vi "Query Temperature.vi"(8 "error in (no error)":errorcluster, 11 "VISA resource name":refnum<visa-resource-name>) -> (0 "error out":errorcluster, 1 "Ch2 Temp (C)":i32(slide) scale=0.0..150.0, 2 "Ch1 Temp (C)":i32(slide) scale=0.0..150.0, 3 "VISA resource name out":refnum<visa-resource-name>, 4 "IC Temp (C)":i32(slide) scale=0.0..150.0, 5 "Temps":T1 {"IC Temp (C)" scale=0.0..150.0; "Ch2 Temp (C)" scale=0.0..150.0; "Ch1 Temp (C)" scale=0.0..150.0})   [LabVIEW 2012, in "Roboteq.lvlib"]
uses:
  Roboteq.lvlib
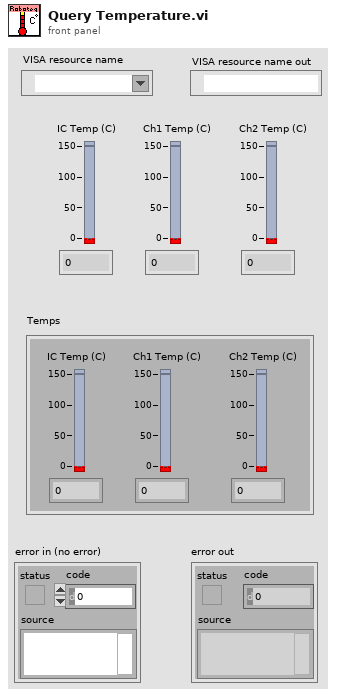
[diagram p1: front panel]
types:
  T1 = cluster{"Ch1 Temp (C)":i32, "Ch2 Temp (C)":i32, "IC Temp (C)":i32}
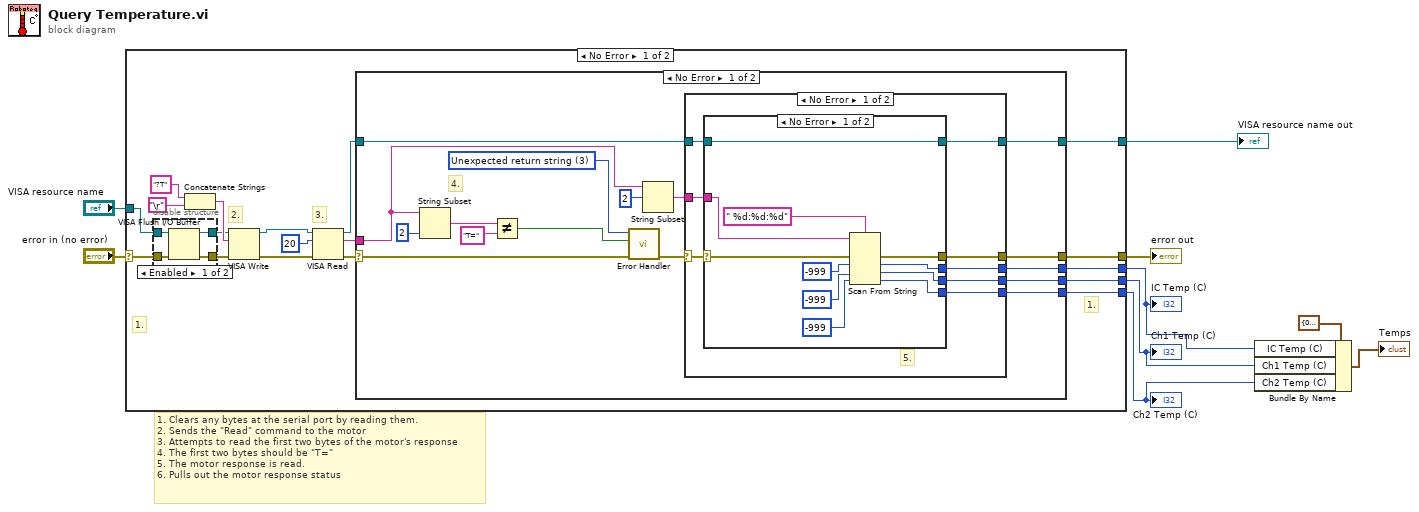
[diagram p0: block diagram]
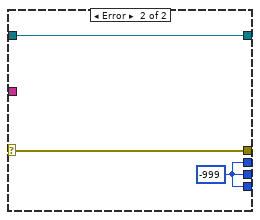
[diagram p3: hidden frame]
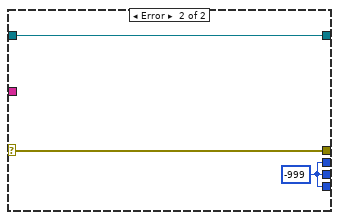
[diagram p4: hidden frame]
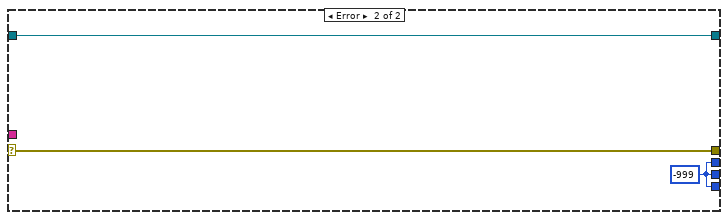
[diagram p5: hidden frame]
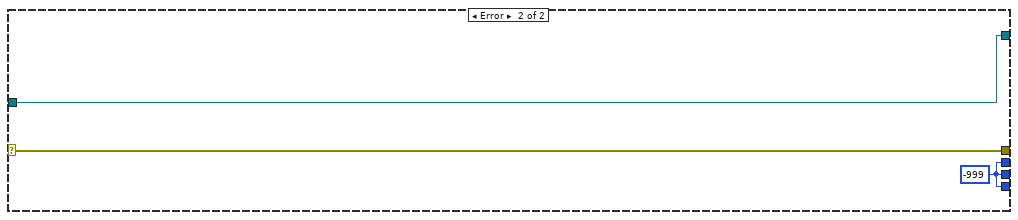
[diagram p6: hidden frame]
diagram:
  # "1. Clears any bytes at the serial port by reading them.\n2. Sends the \"Read\" command to the motor\n3. Attempts to read the first two bytes of the motor's response\n4. The first two bytes should be \"T=\"\n5. The motor response is read.\n6. Pulls out the motor response status"
  n1 = case shown="No Error" "error in (no error)" {
    selector: "error in (no error)" -> [w12 w80]
    tunnel: [w15 w80] -> w8
    tunnel: [w17 w79] -> w2
    tunnel: [w16 w79] -> w1
    tunnel: [w18 w79] -> w3
    tunnel: "VISA resource name" -> [w13 w78]
    tunnel: [w14 w78] -> w6
    frame No Error {
      # "1."
      # "3."
      # "2."
      # "1."
      n2 = disable-structure shown="Enabled" {
        disable-tunnel: w13 -> [w31 w33]
        disable-tunnel: w12 -> [w30 w32]
        disable-tunnel: [w29 w32] -> w11
        disable-tunnel: [w28 w33] -> w10
        frame Enabled {
          n3 = VISA Flush I/O Buffer(VISA resource name=w31, error in (no error)=w30) -> (VISA resource name out=w28:refnum<visa-resource-name>, error out=w29:errorcluster)  [unwired: 1 in]
        }
        frame Disabled {
        }
      }
      n4 = Concatenate Strings("?T" ("string"), "\r") -> (w26:string)
      n5 = VISA Write(VISA resource name=w10, write buffer=w26, error in (no error)=w11) -> (VISA resource name out=w23:refnum<visa-resource-name>, error out=w22:errorcluster)  [unwired: 1 out]
      n6 = VISA Read(VISA resource name=w23, byte count=u32 20, error in (no error)=w22) -> (VISA resource name out=w20:refnum<visa-resource-name>, read buffer=w19:string, error out=w21:errorcluster)  [unwired: 1 out]
      n7 = case shown="No Error" w21 {
        selector: w21 -> [w45 w77]
        tunnel: w19 -> [w36 _]
        tunnel: [w47 w77] -> w15
        tunnel: w20 -> [w49 w76]
        tunnel: [w48 w76] -> w14
        tunnel: [w41 w75] -> w18
        tunnel: [w40 w75] -> w17
        tunnel: [w39 w75] -> w16
        frame No Error {
          w42 = u16 3 items=["Scan timeout"=1, "Invalid motor checksum"=2, "Unexpected return string"=3, "Invalid address range"=4] ("Error type")
          # "4."
          n8 = String Subset(string=w36, length (rest)=2 ("length (rest)")) -> (substring=w35:string)  [unwired: 1 in]
          n9 = Not Equal?(x=w35, y="T=" ("string")) -> (x != y?=w44:bool)
          n10 = call "Error Handler.vi"("error in (no error)"=w45, "Error? (no error)"=w44, "Error type"=w42) -> ("error out"=w46:errorcluster)  [unwired: 8 in]
          n11 = String Subset(string=w36, offset (0)=2 ("length (rest)")) -> (substring=w34:string)  [unwired: 1 in]
          n12 = case shown="No Error" w46 {
            selector: w46 -> [w51 w73]
            tunnel: w49 -> [w52 w74]
            tunnel: [w56 w74] -> w48
            tunnel: [w57 w73] -> w47
            tunnel: [w55 w72] -> w41
            tunnel: [w54 w72] -> w40
            tunnel: [w53 w72] -> w39
            tunnel: w34 -> [w50 _]
            frame No Error {
              # "5."
              n13 = case shown="No Error" w51 {
                selector: w51 -> [w64 w71]
                tunnel: w50 -> [w63 _]
                tunnel: [w62 w71] -> w57
                tunnel: [w68 w70] -> w56
                tunnel: w52 -> [w68 w70]
                tunnel: [w59 w69] -> w55
                tunnel: [w61 w69] -> w54
                tunnel: [w60 w69] -> w53
                frame No Error {
                  n14 = Scan From String(format string=" %d:%d:%d", input string=w63, error in=w64, default 1=-999 ("default value 1"), default 2=-999 ("default value 1"), default 3=-999 ("default value 1")) -> (error out=w62:errorcluster, output 1=w59:i32, output 2=w61:i32, output 3=w60:i32)  [unwired: 1 in, 2 out]
                }
                frame Error {
                  w69 = -999 ("main battery\nvoltage (V)")
                }
              }
            }
            frame Error {
              w72 = -999 ("main battery\nvoltage (V)")
            }
          }
        }
        frame Error {
          w75 = -999 ("main battery\nvoltage (V)")
        }
      }
    }
    frame Error {
      w79 = -999 ("main battery\nvoltage (V)")
    }
  }
  "VISA resource name out" <- w6
  "error out" <- w8
  "Ch1 Temp (C)" <- w2
  "Ch2 Temp (C)" <- w1
  "IC Temp (C)" <- w3
  n15 = Bundle By Name(cluster=T1 {"Ch1 Temp (C)"=0, "Ch2 Temp (C)"=0, "IC Temp (C)"=0} ("Temps"), "IC Temp (C)"=w3, "Ch1 Temp (C)"=w2, "Ch2 Temp (C)"=w1) -> (→"Temps":T1)
